vi "avgdata.vi"(0 "object in":refnum<class "212format_work.lvclass">, 1 "in":T2, 5 "error in (no error)":errorcluster) -> (14 "object out":refnum<class "212format_work.lvclass">, 15 "out":T1, 19 "error out":errorcluster)   [LabVIEW 2016, in "212format_work.lvclass"]
uses:
  212format_work.lvclass
  212format_work.lvclass/212format_work.ctl
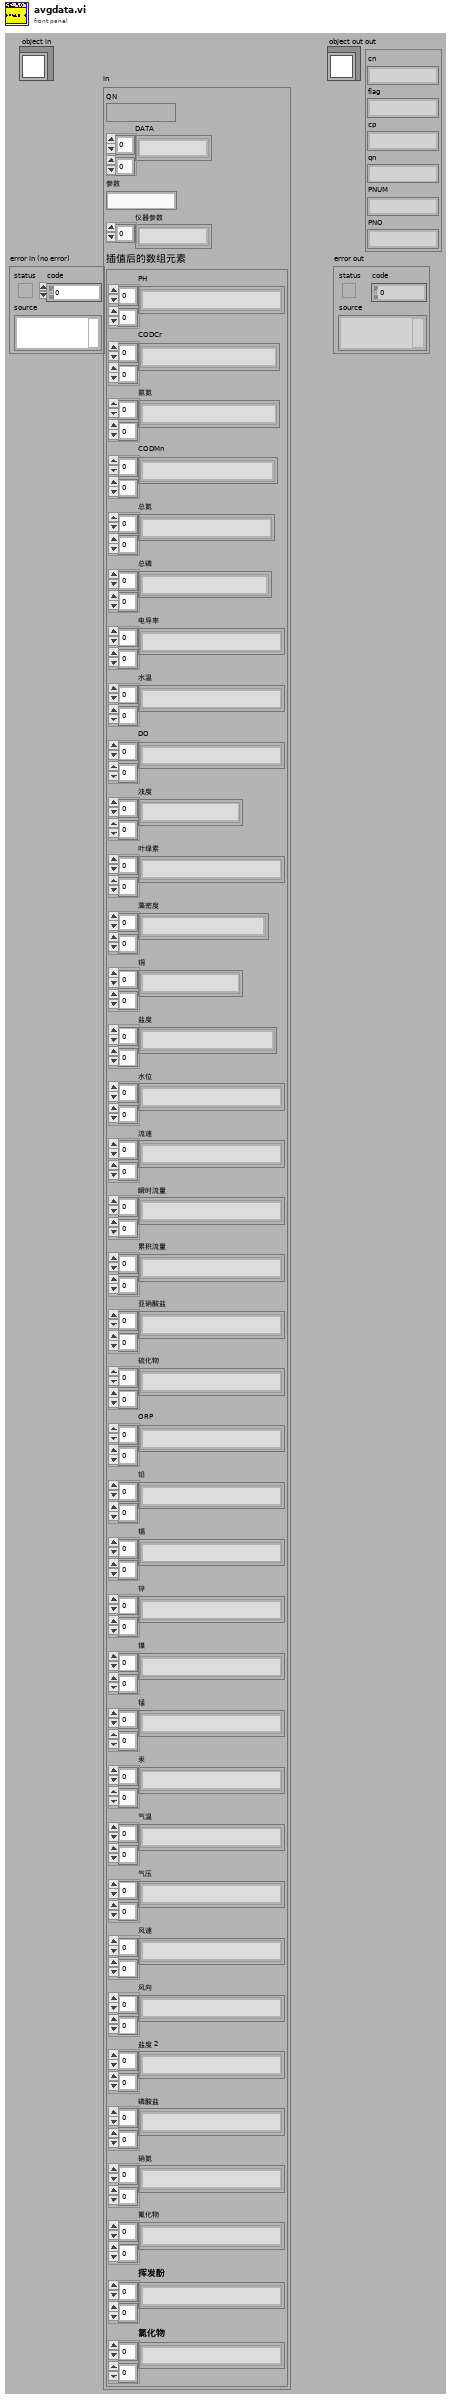
[diagram p1: front panel]
types:
  T1 = cluster{"cn":string, "flag":string, "cp":string, "qn":string, "PNUM":string, "PNO":string}
  T2 = cluster{"QN":string, "DATA":string[][], "参数":string, "仪器参数":string[], "插值后的数组元素":cluster{"PH":string[][], "CODCr":string[][], "氨氮":string[][], "CODMn":string[][], "总氮":string[][], "总磷":string[][], "电导率":string[][], "水温":string[][], "DO":string[][], "浊度":string[][], "叶绿素":string[][], "藻密度":string[][], "铜":string[][], "盐度":string[][], "水位":string[][], "流速":string[][], "瞬时流量":string[][], "累积流量":string[][], "亚硝酸盐":string[][], "硫化物":string[][], "ORP":string[][], "铅":string[][], "镉":string[][], "锌":string[][], "镍":string[][], "锰":string[][], "汞":string[][], "气温":string[][], "气压":string[][], "风速":string[][], "风向":string[][], "盐度 2":string[][], "磷酸盐":string[][], "硝氮":string[][], "氟化物":string[][], "挥发酚":string[][], "氯化物":string[][]}}
  T3 = enum16{"formattime", "formatminute", "formathour"}
  T4 = enum16{"小时数据", "实时数据", "平行样测试", "集成干预测试", "加标回收测试", "核查数据", "空白零点跨度数据", "提取小时数据", "提取实时数据", "操作日志", "仪器参数", "3090仪器参数", "提取仪器参数", "报警信息"}
  T5 = typedef "212format_work.lvclass/interdata控件.ctl" = cluster{"数据发送协议":enum16{"2005-212协议", "2017-212协议"}, "枚举":enum16{"返回请求应答", "上传数据", "返回执行结果"}, "系统编码ST":string, "主动上报数据中":bool, "数据组合发送":bool, "地表水/污染源":bool, "应用环境":enum16{"STD", "GB212"}}
  T6 = typedef "212format_work.lvclass/data控件.ctl" = cluster{"选择发送的参数":string, "插值后的数组元素":cluster{"PH":string[][], "CODCr":string[][], "氨氮":string[][], "CODMn":string[][], "总氮":string[][], "总磷":string[][], "电导率":string[][], "水温":string[][], "DO":string[][], "浊度":string[][], "叶绿素":string[][], "藻密度":string[][], "铜":string[][], "盐度":string[][], "水位":string[][], "流速":string[][], "瞬时流量":string[][], "累积流量":string[][], "亚硝酸盐":string[][], "硫化物":string[][], "ORP":string[][], "铅":string[][], "镉":string[][], "锌":string[][], "镍":string[][], "锰":string[][], "汞":string[][], "气温":string[][], "气压":string[][], "风速":string[][], "风向":string[][], "盐度 2":string[][], "磷酸盐":string[][], "硝氮":string[][], "氟化物":string[][], "挥发酚":string[][], "氯化物":string[][]}, "register values":u16[], "columns输出":string[], "环境参数":string[][], "仪器编码":string, "实时数据发送间隔":u32, "实时数据参数":string, "参数系数簇":cluster{"CODMn":dbl, "CODCr":dbl, "DO":dbl, "铜":dbl, "PH":dbl, "氨氮":dbl, "比电导率":dbl, "水温":dbl, "COD":dbl, "浊度":dbl, "总氮":dbl, "总磷":dbl, "叶绿素a":dbl, "藻密度":dbl, "水位":dbl, "流速":dbl, "瞬时流量":dbl, "累积流量":dbl, "亚硝酸盐":dbl, "硫化物":dbl, "ORP":dbl, "铅":dbl, "镉":dbl, "锌":dbl, "镍":dbl, "锰":dbl, "汞":dbl, "气温":dbl, "气压":dbl, "风速":dbl, "风向":dbl, "盐度":dbl, "磷酸盐":dbl, "硝氮":dbl, "氟化物":dbl, "挥发酚":dbl, "氯化物":dbl}, "因子编码簇":cluster{"CODMn":string, "CODCr":string, "DO":string, "铜":string, "PH":string, "氨氮":string, "比电导率":string, "水温":string, "COD":string, "浊度":string, "总氮":string, "总磷":string, "叶绿素a":string, "藻密度":string, "水位":string, "流速":string, "瞬时流量":string, "累积流量":string, "亚硝酸盐":string, "硫化物":string, "ORP":string, "铅":string, "镉":string, "锌":string, "镍":string, "锰":string, "汞":string, "气温":string, "气压":string, "风速":string, "风向":string, "盐度":string, "磷酸盐":string, "硝氮":string, "氟化物":string, "挥发酚":string, "氯化物":string}, "小时数据发送次数":i32, "读取试剂余量的值":u16[], "参数编码":string, "数据数组大小":i32, "总包数":i32, "当前包号":i32, "columns":string[], "剖面多参数":string[][], "分包标准":i32}
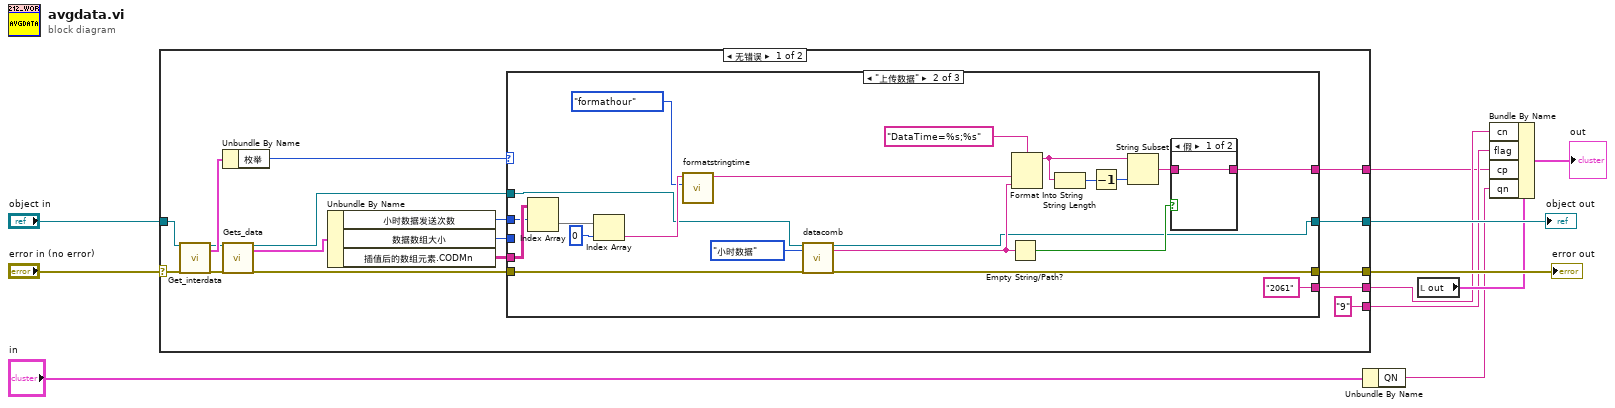
[diagram p0: block diagram]
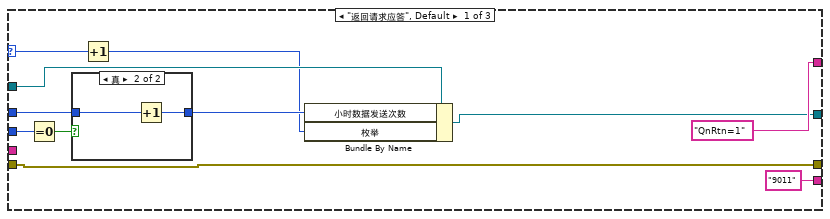
[diagram p2: hidden frame]
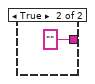
[diagram p4: hidden frame]
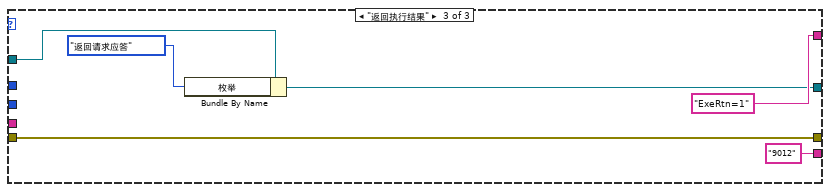
[diagram p5: hidden frame]
diagram:
  n1 = case shown="无错误" "error in (no error)" {
    selector: "error in (no error)" -> [w14 w73]
    tunnel: [w12 w73] -> w10
    tunnel: [w16 w72] -> w8
    tunnel: "object in" -> [w28 w72]
    tunnel: [w25 _] -> w3
    tunnel: ["9" ("ST") _] -> w2
    tunnel: [w23 _] -> w1
    frame No Error {
      n2 = call-dynamic "Get_interdata.vi"("object in"=w28, "error in (no error)"=w14) -> ("object out"=w22:refnum<class "212format_work.lvclass">, "interdata"=w27:T5, "error out"=w21:errorcluster)  [unwired: 15 in]
      n3 = Unbundle By Name(w27) -> ("枚举"=w26:enum16{"返回请求应答", "上传数据", "返回执行结果"})
      n4 = call-dynamic "Gets_data.vi"("object in"=w22, "error in (no error)"=w21) -> ("object out"=w17:refnum<class "212format_work.lvclass">, "data"=w20:T6, "error out"=w13:errorcluster)  [unwired: 15 in]
      n5 = Unbundle By Name(w20) -> ("小时数据发送次数"=w18:i32, "数据数组大小"=w19:i32, "插值后的数组元素.CODMn"=w15:string[][])
      n6 = case shown="\"上传数据\"" w26 {
        selector: w26 -> [w32 _ _]
        tunnel: ["9011" ("CN") "2061" ("CN") "9012" ("CN")] -> w25
        tunnel: ["QnRtn=1" w45 "ExeRtn=1"] -> w23
        tunnel: w17 -> [w37 w50 w69]
        tunnel: w19 -> [w36 _ _]
        tunnel: w18 -> [w34 w48 _]
        tunnel: [w30 w46 w67] -> w16
        tunnel: w15 -> [_ w49 _]
        tunnel: w13 -> [w29 w47 w66]
        tunnel: [w29 w44 w66] -> w12
        frame "返回请求应答", Default {
          n7 = Equal To 0?(x=w36) -> (x = 0?=w35:bool)
          n8 = case shown="真" w35 {
            tunnel: w34 -> [w40 w42]
            tunnel: [w40 w41] -> w33
            frame False {
            }
            frame True {
              n9 = Increment(x=w42) -> (x+1=w41:i32)
            }
          }
          n10 = Increment(x=w32) -> (x+1=w31:enum16{"返回请求应答", "上传数据", "返回执行结果"})
          n11 = Bundle By Name(cluster=w37, "小时数据发送次数"=w33, "枚举"=w31) -> (w30:refnum<class "212format_work.lvclass">)
        }
        frame "上传数据" {
          n12 = Index Array(array=w49, index (row)=w48) -> (element=w61:string[])  [unwired: 1 in]
          n13 = Index Array(array=w61, index=0 ("索引")) -> (element=w59:string)
          n14 = call "formatstringtime.vi"("枚举"=T3."formathour", "字符串"=w59) -> ("result string"=w53:string)  [unwired: 9 in]
          n15 = call-dynamic "datacomb.vi"("object in"=w50, "枚举"=T4."小时数据", "error in (no error)"=w47) -> ("object out"=w46:refnum<class "212format_work.lvclass">, "字符串"=w52:string, "error out"=w44:errorcluster)  [unwired: 14 in]
          n16 = Empty String/Path?(string/path=w52) -> (empty?=w54:bool)
          n17 = Format Into String(format string="DataTime=%s;%s", w53, w52) -> (resulting string=w51:string)  [unwired: 2 in, 1 out]
          n18 = String Length(string=w51) -> (length=w56:i32)
          n19 = Decrement(x=w56) -> (x-1=w57:i32)
          n20 = String Subset(string=w51, length (rest)=w57) -> (substring=w58:string)  [unwired: 1 in]
          n21 = case shown="假" w54 {
            tunnel: [w64 ""] -> w45
            tunnel: w58 -> [w64 _]
            frame False {
            }
            frame True {
            }
          }
        }
        frame "返回执行结果" {
          n22 = Bundle By Name(cluster=w69, "枚举"=enum16{"返回请求应答", "上传数据", "返回执行结果"}."返回请求应答" ("interdata.枚举")) -> (w67:refnum<class "212format_work.lvclass">)
        }
      }
    }
    frame Error {
    }
  }
  "error out" <- w10
  "object out" <- w8
  n23 = Unbundle By Name("in") -> ("QN"=w4:string)
  n24 = local read "out"() -> (w7:T1)
  n25 = Bundle By Name(cluster=w7, "cn"=w3, "flag"=w2, "cp"=w1, "qn"=w4) -> (→"out":T1)
